vi "DT_Triangle Manager_Add Edge_Single Side.vi"(5 "left bottom tri":i32, 7 "left top tri":i32, 8 "right point":i32, 9 "left point":i32, 10 "next triangle in":i32, 11 "Triangles In":i32[][](array[numeric])) -> (2 "next triangle out":i32, 3 "Triangles Out":i32[][](array[numeric]))   [LabVIEW 2017, in "NI_AAL_Geometry.lvlib"]
uses:
  <vilib>/Analysis/NI_AAL_Geometry.lvlib
  <vilib>/Analysis/geometry.llb/DT_Triangle Manager_Get Ghost Point.vi
  <vilib>/Analysis/geometry.llb/DT_Triangle Manager_Get Oppo Point.vi
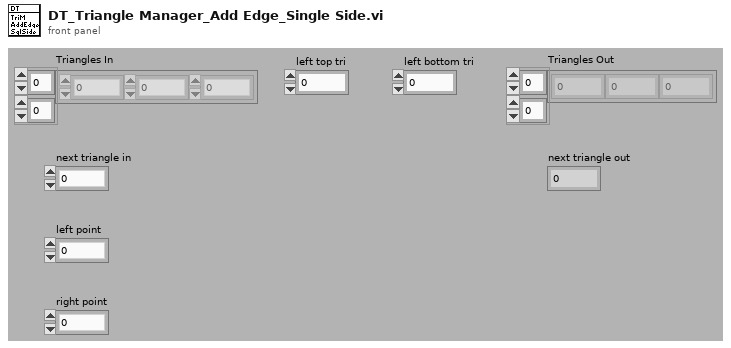
[diagram p1: front panel]
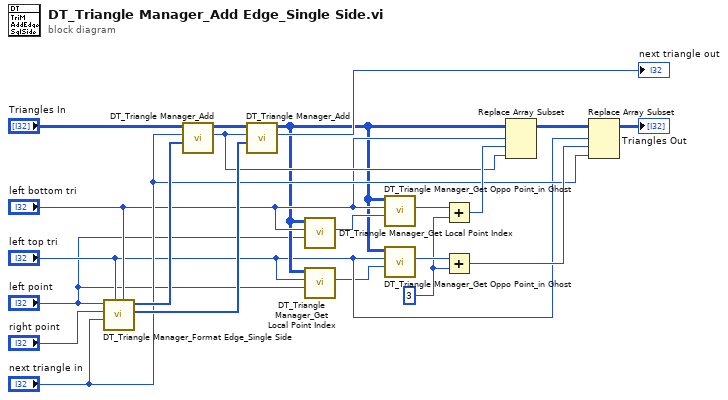
[diagram p0: block diagram]
diagram:
  w11 = 3 ("y")
  n1 = call <vilib>:"DT_Triangle Manager_Format Edge_Single Side.vi"("left bottom tri"="left bottom tri", "left top tri"="left top tri", "start triangle"="next triangle in", "right point"="right point", "left point"="left point") -> ("Second Triangle"=w17:i32[], "First Triangle"=w18:i32[])  [unwired: 5 out]
  n2 = call <vilib>:"DT_Triangle Manager_Add.vi"("Triangle"=w18, "next triangle in"="next triangle in", "Triangles In"="Triangles In") -> ("next triangle out"=w8:i32, "Triangles Out"=w20:i32[][])  [unwired: 7 out]
  n3 = call <vilib>:"DT_Triangle Manager_Add.vi"("Triangle"=w17, "next triangle in"=w8, "Triangles In"=w20) -> ("next triangle out"=→"next triangle out":i32, "Triangles Out"=w4:i32[][])  [unwired: 7 out]
  n4 = call <vilib>:"DT_Triangle Manager_Get Local Point Index.vi"("global idx"="left point", "triangle"="left bottom tri", "Triangles"=w4) -> ("local idx"=w6:i32)  [unwired: 8 out]
  n5 = call <vilib>:"DT_Triangle Manager_Get Local Point Index.vi"("global idx"="left point", "triangle"="left top tri", "Triangles"=w4) -> ("local idx"=w1:i32)  [unwired: 8 out]
  n6 = call <vilib>:"DT_Triangle Manager_Get Oppo Point_in Ghost.vi"("point idx"=w6, "triangle"="left bottom tri", "Triangles"=w4) -> ("opposite point idx"=w13:i32)  [unwired: 8 out]
  n7 = call <vilib>:"DT_Triangle Manager_Get Oppo Point_in Ghost.vi"("point idx"=w1, "triangle"="left top tri", "Triangles"=w4) -> ("opposite point idx"=w12:i32)  [unwired: 8 out]
  n8 = Add(x=w13, y=w11) -> (x+y=w10:i32)
  n9 = Add(x=w12, y=w11) -> (x+y=w9:i32)
  n10 = Replace Array Subset(array=w4, new element=w8, index (row)="left bottom tri", index (col)=w10) -> (w15:i32[][])
  n11 = Replace Array Subset(array=w15, new element="next triangle in", index (row)="left top tri", index (col)=w9) -> (→"Triangles Out":i32[][])
